vi "Overlay.vi"(8 "error in (no error)":errorcluster, 10 "Image In":T1, 11 "Overlay Base in":refnum<class "Analyze Compound Results Base.lvclass">) -> (0 "error out":errorcluster, 2 "Image out":T1, 3 "Overlay Base out":refnum<class "Analyze Compound Results Base.lvclass">)   [LabVIEW 2020, in "Analyze Compound Results Base.lvclass"]
uses:
  Analyze Compound Results Base.lvclass
  <vilib>/vision/Image Controls.llb/IMAQ Image.ctl
  Analyze Compound Results Base.lvclass/Analyze Compound Results Base.ctl
  Results Base/Analyze Results Base.lvclass
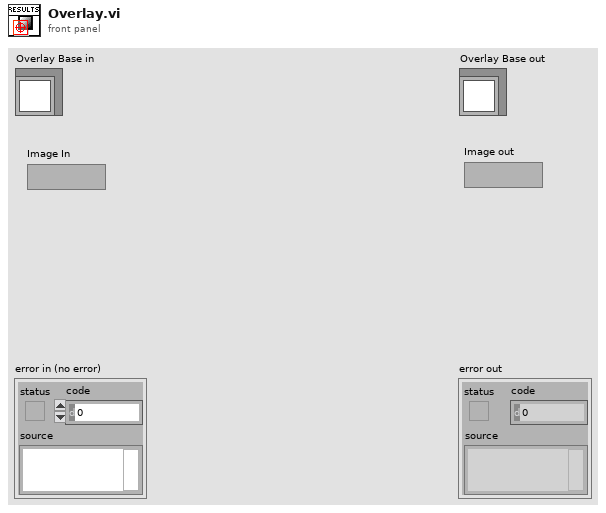
[diagram p1: front panel]
types:
  T1 = typedef "IMAQ Image.ctl" = refnum<image>
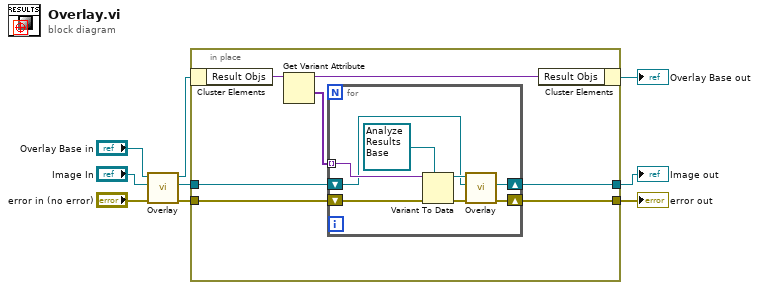
[diagram p0: block diagram]
diagram:
  n1 = call-parent "Overlay.vi"("error in (no error)"="error in (no error)", "Image In"="Image In", "Overlay Base in"="Overlay Base in") -> ("error out"=w4:errorcluster, "Image out"=w2:T1, "Overlay Base out"=w6:refnum<class "Analyze Compound Results Base.lvclass">)  [unwired: 6 in]
  n2 = in-place {
    in-place-border: w2 -> [w13]
    in-place-border: w4 -> [w12]
    in-place-border: [w11] -> w3
    in-place-border: [w10] -> w1
    n3 = in-place-cluster #1(w6) -> ("Result Objs"=w16:variant)
    n4 = Get Variant Attribute(Variant=w16) -> (duplicate Variant=w15:variant, values=w14:variant[])  [unwired: 3 in, 2 out]
    n5 = for {
      tunnel: w14 -> [w24] mode=indexing
      shift-right: [w19] -> w10
      shift-left: w13 -> [w21]
      shift-right: [w18] -> w11
      shift-left: w12 -> [w20]
      n6 = Variant To Data(error in=w20, type=refnum<class "Analyze Results Base.lvclass"> refnum ("Analyze Results Base.lvclass"), Variant=w24) -> (data=w22:refnum<class "Analyze Results Base.lvclass">, error out=w17:errorcluster)
      n7 = call-dynamic "Overlay.vi"("error in (no error)"=w17, "Image In"=w21, "Overlay Base in"=w22) -> ("error out"=w18:errorcluster, "Image out"=w19:T1)  [unwired: 6 in, 1 out]
    }
    n8 = in-place-cluster #1("Result Objs"=w15) -> (→"Overlay Base out":refnum<class "Analyze Compound Results Base.lvclass">)
  }
  "error out" <- w3
  "Image out" <- w1
